vi "BDD READWRIGHT.vi"(7 "Read?":bool, 8 "errin":errorcluster, 10 "DSN name":string, 11 "Instruction":string) -> (0 "error out":errorcluster, 3 "Array":string[][](array[string]))   [LabVIEW 2020]
uses:
  <vilib>/addons/database/NI_Database_API.lvlib
  <vilib>/addons/database/Connection.llb/DB Tools Open Connec (String).vi
  <vilib>/addons/database/Connection.llb/Conn Execute.vi
  <vilib>/addons/database/Recordset.llb/Rec Destroy - Connection.vi
  <vilib>/addons/database/Recordset.llb/Rec Fetch Recordset Data (R).vi
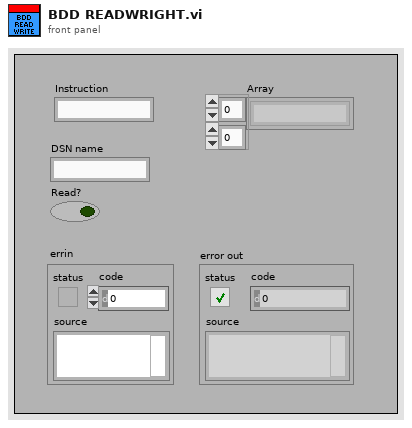
[diagram p1: front panel]
types:
  T1 = typedef "NI_Database_API.lvlib/Conn ObjectReference.ctl" = refnum<k1>
  T2 = typedef "NI_Database_API.lvlib/Rec ObjectReference.ctl" = refnum<k1>
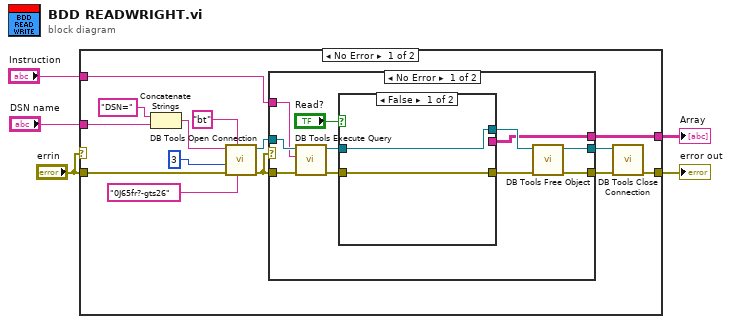
[diagram p0: block diagram]
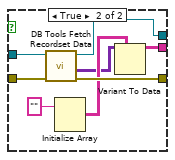
[diagram p2: hidden frame]
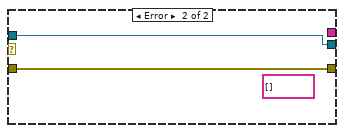
[diagram p3: hidden frame]
diagram:
  n1 = case shown="No Error" "errin" {
    tunnel: "Instruction" -> [w19 _]
    tunnel: [w18 _] -> w4
    tunnel: "DSN name" -> [w15 _]
    tunnel: [w12 w43] -> w2
    tunnel: "errin" -> [w6 w43]
    frame No Error {
      n2 = Concatenate Strings("DSN=" ("password"), w15) -> (w17:string)
      n3 = call-poly <vilib>:"DB Tools Open Connection.vi"("password"="0J65fr?-gts26", "userID"="bt", "error in (no error)"=w6, "connection timeout (15)"=3, "connection information"=w17) -> ("error out"=w13:errorcluster, "connection reference"=w9:T1)  [unwired: 3 in]
      n4 = case shown="No Error" w13 {
        tunnel: w13 -> [w30 w42]
        tunnel: w9 -> [w28 w41]
        tunnel: [w24 w42] -> w10
        tunnel: [w23 w41] -> w11
        tunnel: [w22 _] -> w18
        tunnel: w19 -> [w21 _]
        frame No Error {
          n5 = call-poly <vilib>:"DB Tools Execute Query.vi"("error in (no error)"=w30, "SQL query"=w21, "connection reference"=w28) -> ("error out"=w29:errorcluster, "recordset reference"=w27:T2)  [unwired: 5 in]
          n6 = case shown="False" "Read?" {
            tunnel: w29 -> [w32 w40]
            tunnel: w27 -> [w31 w39]
            tunnel: [w31 w38] -> w26
            tunnel: [w32 w37] -> w25
            tunnel: [_ w33] -> w22
            frame False {
            }
            frame True {
              n7 = call-poly <vilib>:"DB Tools Fetch Recordset Data.vi"("error in (no error)"=w40, "recordset reference"=w39) -> ("error out"=w37:errorcluster, "recordset data"=w34:variant[][], "recordset reference out"=w38:T2)  [unwired: 3 in]
              n8 = Initialize Array("") -> (w35:string[][])  [unwired: 2 in]
              n9 = Variant To Data ("Variant en donnée")(type=w35, Variant=w34) -> (data=w33:string[][])  [unwired: 1 in, 1 out]
            }
          }
          n10 = call-poly <vilib>:"DB Tools Free Object.vi"("error in (no error)"=w25, "recordset reference"=w26) -> ("error out"=w24:errorcluster, "connection reference"=w23:T1)  [unwired: 8 in]
        }
        frame Error {
          (unwired) string[] []
        }
      }
      n11 = call <vilib>:"DB Tools Close Connection.vi"("error in (no error)"=w10, "connection reference"=w11) -> ("error out"=w12:errorcluster)  [unwired: 5 in]
    }
    frame Error {
    }
  }
  "Array" <- w4
  "error out" <- w2
